vi "SciScan GALVO.vi"(11 "System type (Default - Standalone)":T1(ring)) -> ()   [LabVIEW 2012]
doc: "SciScan 1.1f2 160418"
uses:
  Custom Controls/Laser power 2 dial.ctl
  Custom Controls/Ch selector.ctl
  Custom Controls/MAIN Image panel tab Control type def.ctl
  Custom Controls/scan mode main settings tab.ctl
  Custom Controls/speed mode type def.ctl
  Custom Controls/pixel resolution enum.ctl
  Custom Controls/advanced settings inner tab CTL.ctl
  Custom Controls/Laser power 1 dial.ctl
  Custom Controls/Histogram tab.ctl
  Custom Controls/file format type def.ctl
  Custom Controls/experiment type.ctl
  Custom Controls/display palette control.ctl
  Custom Controls/PositionSaveMod.ctl
  Custom Controls/trigger enum.ctl
  HFG/Custom Controls and Typedefs/HFG Commands.ctl
  CommonResource VIs/Timing/Timer Commands.ctl
  HFG/SubVIs/Broken Chain FGV Command.ctl
  Plugins/Macro Module/Macro Rule/subVIs/MacroRules_FGV_Commands.ctl
  Plugins/Macro Module/Macro Rule/subVIs/MacroErrorsFGV_Commands.ctl
  <vilib>/event_ctls.llb/lveventtype.ctl
  INI/settingsIO/Settings IO_Commands.ctl
  Plugins/Macro Module/MacroGUI Module/Custom Controls and Typedefs/GFG Variable for IO.ctl
  GFG/GFGnumericGet.vi
  GFG/GFGfpRefGet.vi
  GFG/GFGpathGet.vi
  GFG/GFGstringGet.vi
  GFG/GFG library.lvlib
panel:
  in  "MAIN UI responsive? (F)":bool
  in  "shutterlock":bool caption="LOCK"
  in  "custom step z":bool
  in  "custom step xy":bool
  in  "no of grid lines":dbl(slide) min=0.0 step=1.0 scale=0.0..20.0
  out "grid size":string caption="GRID"
  in  "save prot":bool
  in  "piezo.active":bool
  in  "PositionSaveButton":T2
  in  "reset zoom":bool
  out "Channel 5 large":T3(plugin-control)
  in  "bool.stage.speed":bool=TRUE
  in  "Stage Stop":bool
  in  "step.size.xy":u16(ring)=1 items=["   1"=1, "   2"=2, "   5"=5, "  10"=10, "  20"=20, "  50"=50, "100"=100]
  in  "Y UP":bool
  in  "X LEFT":bool
  in  "Y DOWN":bool
  in  "X RIGHT":bool
  out "String 6":string
  in  "shutter":bool
  in  "x.pixels":i32=256 min=2 max=2048 step=2
  in  "clear prot":bool
  in  "timestamp.prot":bool
  in  "protocol.notes":string caption="notebook"
  in  "Open All\nSettings":bool=TRUE
  in  "step.size.z":u16(ring)=1 items=["    1"=1, "    2"=2, "    5"=5, "  10"=10, "  20"=20, "  50"=50, "100"=100]
  out "frame count":dbl(slide) scale=0.0..30.0
  in  "scan mode main settings":T4
  in  "pixel resolution":T5=enum."512 x 512"
  in  "speed mode":T6=2 items=["extra fast scan", "fast scan", "standard scan", "long exposure"]
  in  "ROTATE":dbl(knob) min=0.0 max=360.0 step=1.0 scale=0.0..360.0 scale format="%#_3g"
  in  "rotate.enable":bool
  in  "ZOOM":dbl(slide)=1.0 min=1.0 max=20.1 step=0.1 scale=1.0..20.0 scale format="%#.1f"
  in  "no. of frames to acquire":i32=10000 min=2 max=2147483646 step=2
  out "x.fov":dbl caption="Field of view    x" format="%#_3p"
  out "y.fov":dbl caption="y" format="%#_3p"
  out "ms.p.line":dbl caption="ms/line" format="%#.2g"
  out "frames.p.sec":dbl caption="frames/s" format="%#.2g"
  out "pixels per line":i32=10000 min=2 max=2147483646 step=2
  out "lines per second":i32=10000 min=2 max=2147483646 step=2
  in  "linescan.y.pixels":i32=256 caption="Lines to display at once" min=2 max=2048 step=2
  in  "no. of lines to acquire":i32=10000 min=2 max=2147483646 step=2
  in  "experiment type":T7="XYT"
  in  "experiment name":string
  in  "root.path":path=path "d:/"
  in  "Objective":u16(ring) items=["Olympus 10x", "Nikon 20x", "Nikon 16x"]
  in  "file format":T8
  out "stack.duration":i32=10 caption="stack.duration (sec)" min=0 max=2147483646 step=2
  in  "add":bool
  in  "clear all":bool
  in  "clear last":bool
  in  "move to z.stack.\nstart plane":bool
  in  "start z.stack":bool
  in  "frames.per.plane":i32=10000 min=2 step=2
  in  "z.spacing":dbl=1.0 caption="z.spacing (um)" min=0.1 step=0.1
  out "no of planes":i32=10 min=0 max=2147483646 step=2
  in  "no.of.cycles.to.scan":dbl=2.0 caption="no.of.volumes" min=1.0 step=1.0
  out "volume rate (in Hz)":dbl=1.0 min=0.0 max=5.5 step=0.1
  in  "frames.per.z.cycle":dbl=4.0 min=4.0 step=2.0
  in  "piezo.mode":bool
  in  "piezo.offset.compensation.seconds":dbl caption="no.of.volumes"
  in  "Z UP":bool
  in  "Z DOWN":bool
  out "String 7":string
  in  "setY":dbl caption="Z-Stepper" format="%#.1f"
  in  "setX":dbl caption="Z-Stepper" format="%#.1f"
  in  "setZ":dbl caption="set" format="%#.1f"
  out "String 4":string
  out "posZ":dbl caption="actual" format="%#.1f"
  out "posX":dbl caption="Z-Stepper" format="%#.1f"
  out "posY":dbl caption="Z-Stepper" format="%#.1f"
  out "String 3":string
  in  "XYZ stage settings slider tab":enum32{" "}(tab)
  in  "LP enable":bool
  out "String 20":string
  in  "set stage speed":bool
  in  "enable virtual XYZ":bool
  out "String 16":string
  in  "set Y to zero":bool
  in  "set X to zero":bool
  in  "set all to zero":bool
  in  "set Z to zero":bool
  out "String 9":string
  in  "reverse x":bool
  in  "reverse y":bool
  in  "reverse z":bool
  out "String 8":string
  in  "PIN Button XYZ stage settings slider tab":bool=TRUE
  in  "QUIT":bool
  in  "Record":bool
  in  "FOCUS":bool
  in  "MAIN Image panels":T9
  out "Channel 1 large":T3(plugin-control)
  out "Channel 2 large":T3(plugin-control)
  out "Channel 3 large":T3(plugin-control)
  out "Channel 4 large":T3(plugin-control)
  out "Channel 1 small":T3(plugin-control)
  out "Channel 2 small":T3(plugin-control)
  out "Channel 4 small":T3(plugin-control)
  out "Channel 3 small":T3(plugin-control)
  in  "Blue Channel (Overlay)":T10 caption="B"
  in  "Green Channel (Overlay)":T10=enum."Ch 1" caption="G"
  in  "Red Channel (Overlay)":T10=enum."Ch 2" caption="R"
  out "RGB overlay":T3(plugin-control)
  in  "ROI channel":T10=enum."Ch 1" caption="Channel"
  out "ROI chart":sgl[][](graph)=[[54.570076, 54.556858]]
  out "ROI Image display":T3(plugin-control)
  in  "zoom to ROI":bool
  in  "move.to.point.ROI":bool
  in  "load coordinates":bool
  in  "confirm line":bool
  in  "channel arb line scan":T10 caption="Channel"
  out "arb line scan display":T3(plugin-control)
  in  "Cancel":bool
  in  "hist/ref slider tab":enum32{" "}(tab)
  in  "PIN Button hist/ref slider tab":bool=TRUE
  in  "Histograms tab":T11
  in  "auto scale\n      CH 1":bool=TRUE caption="auto scale 2"
  in  "Min Max Channel 1":cluster{dbl, dbl}(slide)={0.0, 2047.0} scale=0.0..2047.0 scale format="%#_4g"
  out "Histogram 1":T12(graph)={"Starting Value"=-2007.0, "Incremental Value"=15.7109375, "Histogram"=[]}
  out "String 12":string
  in  "auto scale\n      CH 4":bool=TRUE caption="auto scale 2"
  in  "Min Max Channel 4":cluster{dbl, dbl}(slide)={0.0, 2047.0} scale=0.0..2047.0 scale format="%#_4g"
  out "Histogram 4":T12(graph)
  out "String 15":string
  in  "auto scale\n      CH 3":bool=TRUE caption="auto scale 2"
  in  "Min Max Channel 3":cluster{dbl, dbl}(slide)={0.0, 2047.0} scale=0.0..2047.0 scale format="%#_4g"
  out "Histogram 3":T12(graph)
  out "String 14":string
  in  "auto scale\n      CH 2":bool=TRUE caption="auto scale 2"
  in  "Min Max Channel 2":cluster{dbl, dbl}(slide)={0.0, 2047.0} scale=0.0..2047.0 scale format="%#_4g"
  out "Histogram 2":T12(graph)
  out "String 13":string
  in  "avg type":u16(ring) items=["none", "group avg", "moving avg"]
  in  "avg of":i8=10 min=2 step=1
  in  "display palette":T13
  in  "large histogram":bool caption="Pop-Out"
  in  "laser power slider tab":enum32{"1", " 2"}(tab)
  in  "enable set power max":bool
  in  "set power max":bool
  in  "Laser Power":T14 min=0.0 max=100.0 step=0.5 scale=0.0..100.0 scale format="%3d"
  in  "PIN Button laser power slider tab":bool=TRUE
  in  "enable set power max 2":bool
  in  "set power max 2":bool
  in  "Laser Power 2":T15 caption="Laser Power" min=0.0 max=100.0 step=0.5 scale=0.0..100.0 scale format="%3d"
  in  "PMT slider tab":enum32{""}(tab)
  in  "PMT 2":u16(slide) max=1000 scale=0.0..1000.0
  in  "PMT 1":u16(slide) max=1250 scale=0.0..1000.0
  out "String 5":string
  in  "PMT 4":u16(slide) max=1000 scale=0.0..1000.0
  in  "PMT 3":u16(slide) max=1250 scale=0.0..1000.0
  out "String 18":string
  in  "PIN Button PMT slider tab":bool=TRUE
  in  "advanced settings slider tab":enum32{""}(tab)
  in  "advanced settings inner tab":T16
  in  "pixel.dwell.time.in.sec":dbl=1e-05 min=4e-07 max=1e-05 step=2e-07 format="%#.6p"
  in  "y.pixel.sz":dbl=1e-05 min=1e-09 max=1e-05 step=1e-07 format="%#_3p"
  in  "x.pixel.sz":dbl=1e-05 min=1e-09 max=1e-05 step=1e-07 format="%#_3p"
  in  "y.pixels":i32=512 caption="Y Resolution" min=2 max=2048 step=2
  in  "fill fraction":dbl=60.0 caption="%" min=60.0 max=100.0 step=0.5 format="%_3g"
  in  "nomin.x.pixels":i32=512 caption="X resolution" min=2 max=2048 step=2
  in  "y bidirectional":bool
  in  "x bidirectional":bool=TRUE
  in  "x.voltage":dbl=0.9999999999999999 min=0.0 max=5.5 step=0.1
  in  "y.voltage":dbl=1.0 min=0.0 max=5.5 step=0.1
  in  "y.volt.offset":dbl=-0.2 step=0.1
  in  "x.volt.offset":dbl=-0.2 step=0.1
  in  "voltage.for\nmax.field.of.view":dbl=5.0 min=0.0 max=5.0
  in  "max.field.of.view":dbl=300.0 format="%#_6p"
  in  "x.invert.image":bool
  in  "y.invert.image":bool
  in  "autocorrect.startdelay":bool
  out "pixel.dwell.time.in.ticks":u16=20 min=2 step=1
  out "sample.clock":dbl=5000000.0
  out "ADsamples.per.frame":i32
  in  "Start.Delay":dbl(slide)=1.0 min=1.0 max=10000000.0 step=1.0 scale=1.0..1000.0
  in  "invert.ch.3":bool
  in  "invert.ch.2":bool
  in  "invert.ch.1":bool
  in  "invert.ch.0":bool caption="invert"
  in  "ai.active3":bool
  in  "ai.active2":bool
  in  "ai.active1":bool
  in  "ai.active0":bool caption="active"
  in  "ai.range2":dbl=10.0 min=0.1 max=10.0 step=0.1
  in  "ai.range1":dbl=10.0 min=0.1 max=10.0 step=0.1
  out "ai.string3":string
  out "ai.string2":string
  out "ai.string1":string
  out "ai.string0":string caption="Analog Input"
  in  "ai.range0":dbl=10.0 caption="input range\n      (+/-)" min=0.1 max=10.0 step=0.1
  in  "ai.range3":dbl=10.0 min=0.1 max=10.0 step=0.1
  in  "Pulse\nevery n frames":i32=2 min=1 max=10000 step=1
  in  "Initial delay\n[frames]":dbl=2.0 min=0.1 step=1.0
  in  "pulse.Boolean":bool
  in  "external.start.trigger.enable":bool=TRUE caption="WAIT FOR TRIGGER from external device"
  in  "trigger.enum":T17=enum."trigger off" caption="SEND TRIGGER to external device"
  in  "Initial delay\n[ms]":dbl=2.0 min=0.1 max=170000.0 step=1.0
  in  "Pulse\nduration [ms]":dbl=2.0 min=0.1 step=1.0
  in  "Pulse\nfrequency [Hz]":dbl=2.0 min=0.01 max=10000.0 step=1.0
  in  "abs/rel z pos":enum32{"abs", "rel"}(tab)
  in  "pos  pockels cell PMT Data":dbl[][](array[numeric]) caption="Data" format="%0.1f"
  in  "RELATIVE pos  pockels cell PMT Data":dbl[][](array[numeric]) caption="Data" format="%0.1f"
  in  "PIN Button advanced settings slider tab":bool=TRUE
  in  "SCIENTIFICA Button":bool
  # "to zoom out press and hold Shift"
  # "OFF"
  # "2x2"
  # "4x4"
  # "6x6"
  # "8x8"
  # "10x10"
  # "12x12"
  # "14x14"
  # "16x16"
  # "18x18"
  # "20x20"
  # "abs  pos."
  # "x"
  # "y"
  # "z"
  # "rel pos."
  # "x"
  # "y"
  # "z"
  # "Z Stack parameters"
  # "Z Stack plane management"
  # "zig-zag (leaf scan)"
  # "sawtooth"
  # "Typically, the response lag of piezo positioning is in the millisecond range. Use negative values to compensate for this lag.  Example: -0.015 seconds"
  # "reverse \ndirection"
  # "Zero\nrel. pos."
  # "z"
  # "x"
  # "y"
  # "LP enable"
  # "virtual XYZ"
  # "Press and hold Ctrl to add multiple ROIs"
  # "Average frames (display only)"
  # "frames"
  # "ms \nHz"
  # "X"
  # "Y"
  # "Z"
  # "LASER1"
  # "LASER2"
  # "X"
  # "Y"
  # "Z"
  # "LASER1"
  # "LASER2"
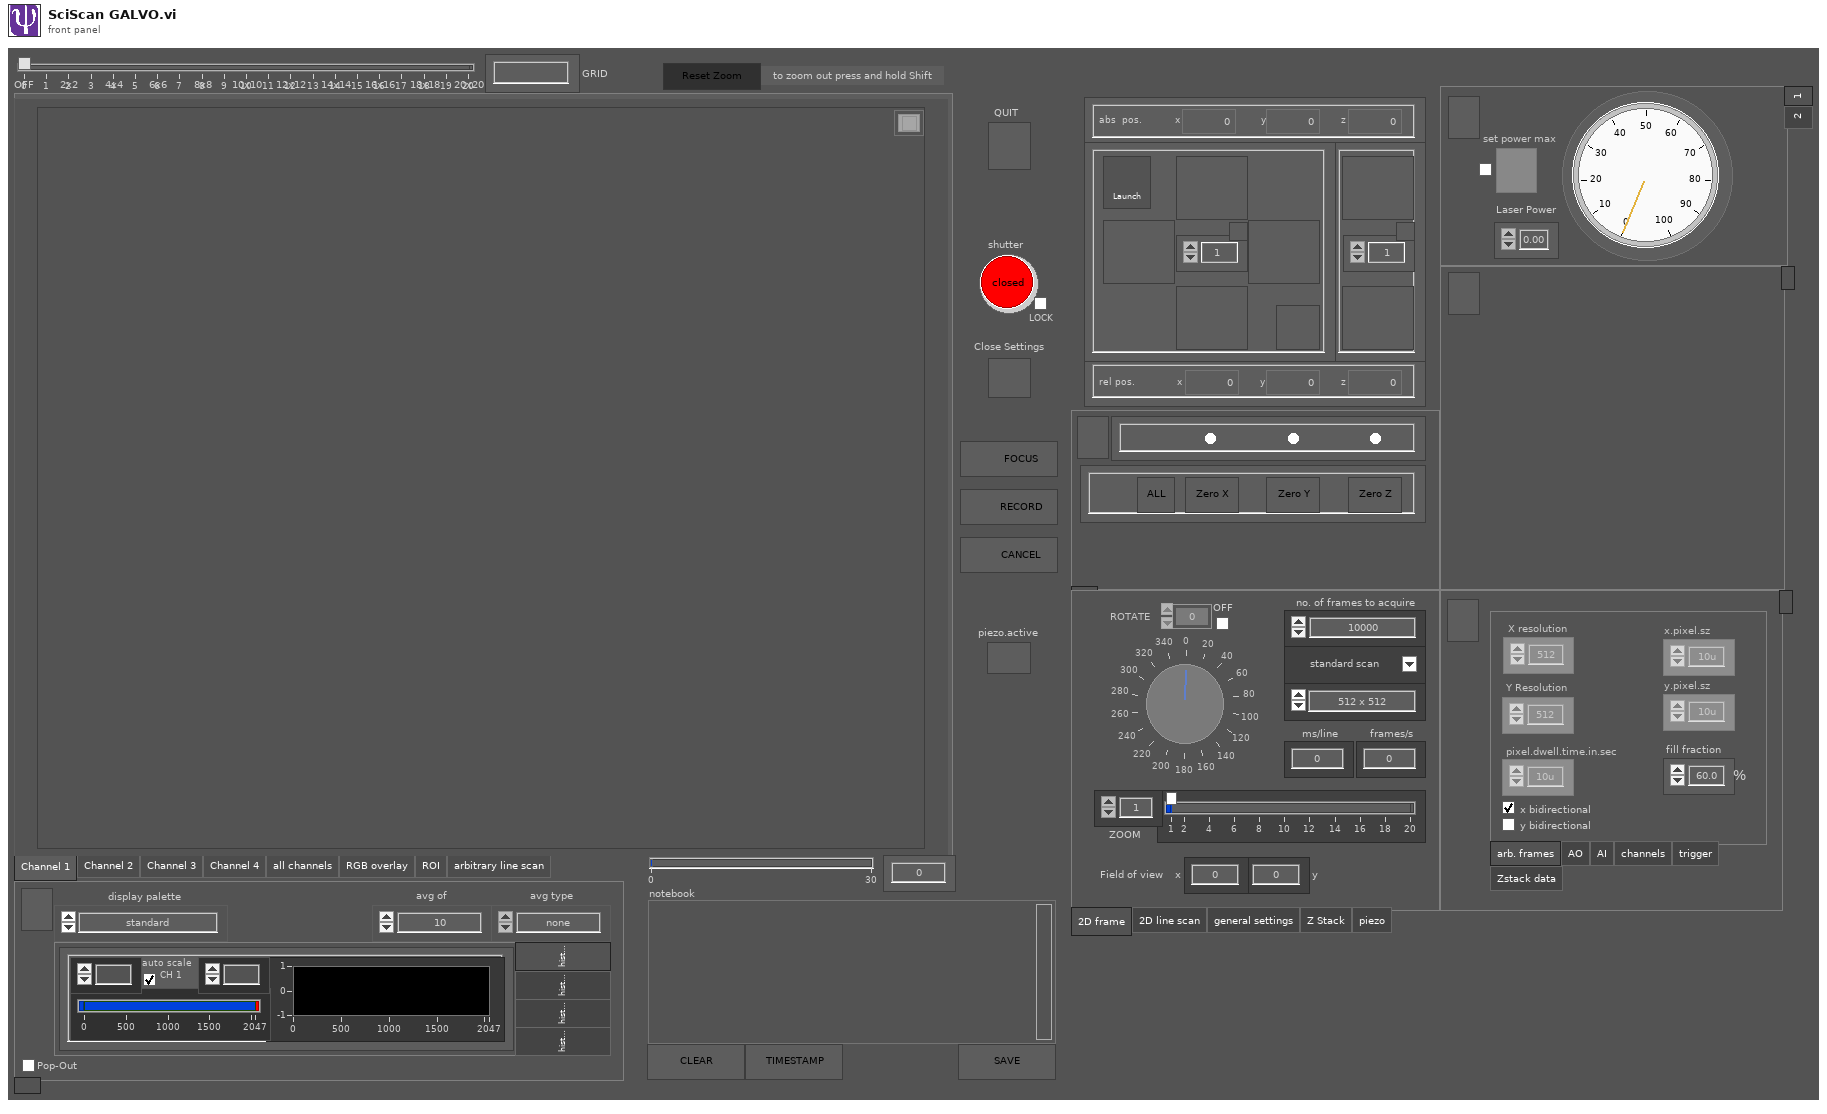
[diagram p1: front panel]
types:
  T1 = enum16{"Standalone Galvo", "Imaging Galvo", "Photostimulation Galvo"}
  T2 = typedef "PositionSaveMod.ctl" = bool
  T3 = typedef "IMAQ Image.ctl" = refnum<image>
  T4 = typedef "scan mode main settings tab.ctl" = enum32{"2D frame", "2D line scan", "general settings", "Z Stack", "piezo"}
  T5 = typedef "pixel resolution enum.ctl" = enum16{"128 x 128", "256 x 128", "256 x 256", "512 x  64", "512 x 128", "512 x 256", "512 x 512", "1024 x 512", "1024 x 1024", "arbitrary"}
  T6 = typedef "speed mode type def.ctl" = u16
  T7 = typedef "experiment type.ctl" = string
  T8 = typedef "file format type def.ctl" = enum16{"16bit raw", "32bit raw", "16bit multi-tiff (interleave)", "16bit multi-tiff (separate)", "16bit multi-tiff (stacked)", "32bit multi-tiff (interleave)", "32bit multi-tiff (separate)", "32bit multi-tiff (stacked)", "16bit tiff series (interleave)", "16bit tiff series (separate)", "16bit tiff series (stacked)", "32bit tiff series (interleave)", "32bit tiff series (separate)", "32bit tiff series (stacked)"}
  T9 = typedef "MAIN Image panel tab Control type def.ctl" = enum32{"Channel 1", "Channel 2", "Channel 3", "Channel 4", "all channels", "RGB overlay", "ROI", "arbitrary line scan"}
  T10 = typedef "Ch selector.ctl" = enum16{"none", "Ch 1", "Ch 2", "Ch 3", "Ch 4"}
  T11 = typedef "Histogram tab.ctl" = enum32{"hist Ch 1", "hist Ch 4", "hist Ch 3", "hist Ch 2"}
  T12 = cluster{"Starting Value":sgl, "Incremental Value":sgl, "Histogram":u32[]}
  T13 = typedef "display palette control.ctl" = enum16{"standard", "high clipping red", "low clipping blue", "high and low clipping", "high / low (full range)"}
  T14 = typedef "Laser power 1 dial.ctl" = dbl
  T15 = typedef "Laser power 2 dial.ctl" = dbl
  T16 = typedef "advanced settings inner tab CTL.ctl" = enum32{"arb. frames", "AO", "AI", "channels", "trigger", "Zstack data"}
  T17 = typedef "trigger enum.ctl" = enum16{"legacy frame pulser PFI4", "continuous pulses", "single pulse", "trigger off"}
  T18 = enum16{"Get Settings Table ", "Read Settings File", "Get Specified Settings"}
  T19 = typedef "MacroErrorsFGV_Commands.ctl" = enum16{"Initialize", "Get Error Array", "Set Error Array"}
  T20 = typedef "MacroRules_FGV_Commands.ctl" = enum16{"Read File", "Get All", "Get Param and Flags"}
  T21 = typedef "Broken Chain FGV Command.ctl" = enum16{"Initialize", "Update VI status", "Get All VI status"}
  T22 = typedef "Timer Commands.ctl" = enum16{"Clear All", "Start", "Pause", "Check Time"}
  T23 = typedef "HFG Commands.ctl" = enum16{"Set", "Get", "Initialize"}
  T24 = enum8{"Enabled", "Disabled", "Disabled and Grayed Out"}
  T25 = typedef "Image Type" = u32
  T26 = cluster{refnum<vi>, refnum<vi>, refnum<vi>, refnum<vi>, refnum<vi>, refnum<vi>, refnum<vi>, refnum<vi>, refnum<vi>, refnum<vi>, refnum<vi>, refnum<vi>}
  T27 = cluster{"New Image":T3, "New Image":T3, "New Image":T3, "New Image":T3, "New Image":T3, "New Image":T3, "New Image":T3, "New Image":T3, "New Image":T3, "New Image":T3, "New Image":T3, "New Image":T3}
  T28 = cluster{"WaveformChartRef":refnum<vi>, "DigitalRef":refnum<vi>, "ArrayRef":refnum<vi>, "TabControlRef":refnum<vi>, "EnumRef":refnum<vi>, "RingRef":refnum<vi>, "BooleanRef":refnum<vi>, "KnobRef":refnum<vi>, "SlideRef":refnum<vi>, "PathRef":refnum<vi>, "StringRef":refnum<vi>, "ComboBox":refnum<vi>, "WaveformGraphRef":refnum<vi>}
  T29 = typedef "lveventtype.ctl" = enum32{"Null", "Timeout", "Annotation Menu Selection", "Annotation Menu Selection?", "App Instance Close", "App Instance Close?", "Autoscale Range Change", "Cell Edit", "Cell Edit?", "Cursor Grab", "Cursor Grab?", "Cursor Menu Selection", "Cursor Menu Selection?", "Cursor Move", "Cursor Release", "Data Change", "Direction Change", "Display State Change", "Drag Ended", "Drag Enter", "Drag Leave", "Drag Over", "Drag Source Update", "Drag Starting", "Drag Starting?", "Drop", "Exec State Change", "Key Down", "Key Down?", "Key Repeat", "Key Repeat?", "Key Up", "Listbox Double Click", "Menu Activation?", "Menu Selection (App)", "Menu Selection? (App)", "Menu Selection (User)", "Mouse Down", "Mouse Down?", "Mouse Enter", "Mouse Leave", "Mouse Move", "Mouse Up", "NI Security User Change (App)", "Pane Size", "Panel Close", "Panel Close?", "Panel Resize", "Plot Attribute Change", "Scale Range Change", "Shortcut Menu Activation?", "Shortcut Menu Selection (App)", "Shortcut Menu Selection? (App)", "Shortcut Menu Selection (User)", "Tree Double Click", "Tree Drag", "Tree Drag?", "Tree Drop", "Tree Drop?", "Tree Item Close", "Tree Item Close?", "Tree Item Open", "Tree Item Open?", "Value Change"}
  T30 = enum32{"Invalid", "Standard", "Closed", "Hidden", "Minimized", "Maximized"}
  T31 = enum32{"Invalid", "Default", "Floating", "Floating/Auto-Hide", "Modal"}
  T32 = typedef "Settings IO_Commands.ctl" = enum16{"Write HW Settings", "Write Config Settings", "Read HW Settings", "Read Config Settings", "Write Line-Scan Settings", "Write Frame-Scan Settings", "Write Z-Stack Settings", "Read Line-Scan Settings", "Read Frame-Scan Settings", "Read Z-Stack Settings", "Read Fast-Z Settings", "Write Fast-Z Settings"}
  T33 = typedef "GFG Variable for IO.ctl" = cluster{"Variable Name":string, "Value (Variant)":variant, "data type":string}
  T34 = enum32{"Page Enabled", "Page Disabled", "Page Disabled & Grayed"}
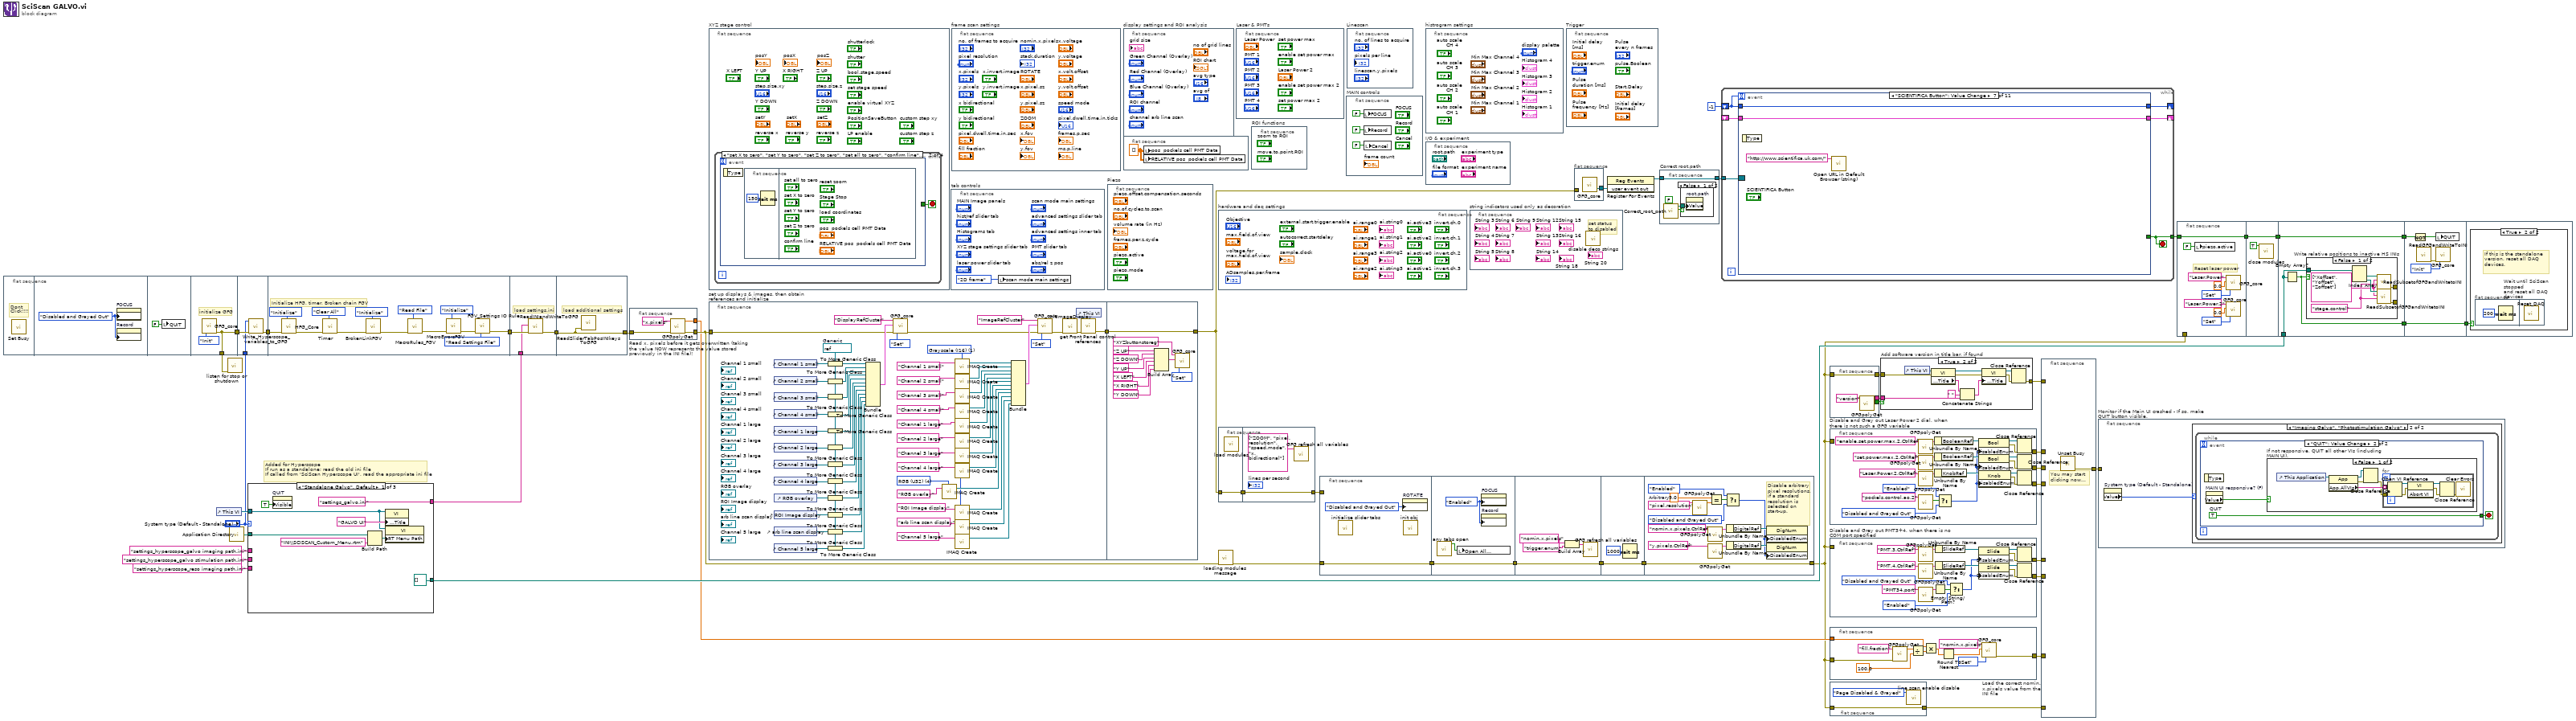
[diagram p0: block diagram]
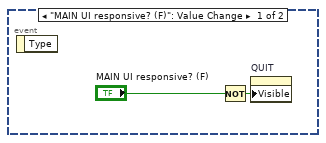
[diagram p3: hidden frame]
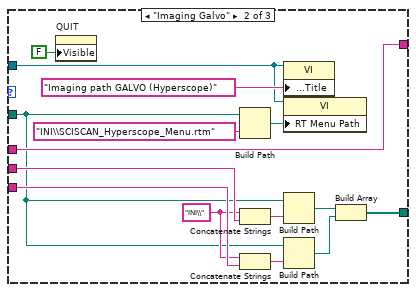
[diagram p6: hidden frame]
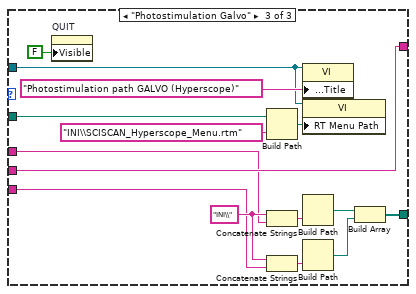
[diagram p7: hidden frame]
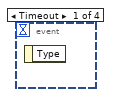
[diagram p9: hidden frame]
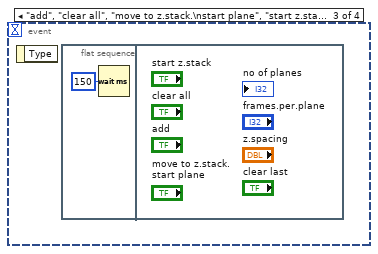
[diagram p10: hidden frame]
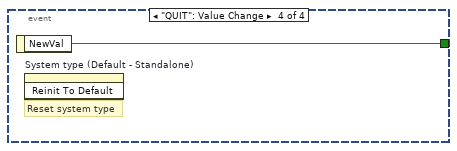
[diagram p11: hidden frame]
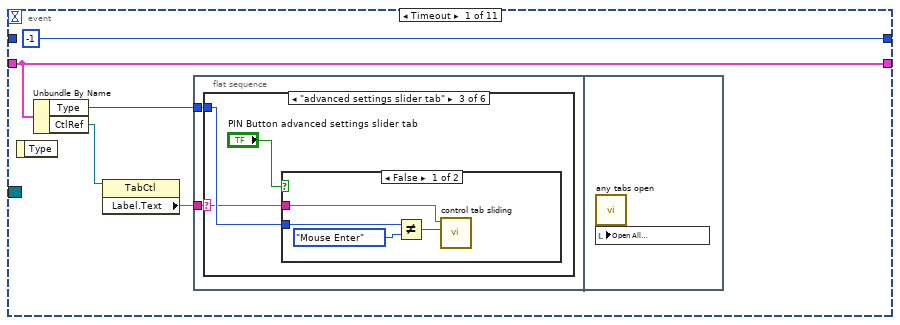
[diagram p14: hidden frame]
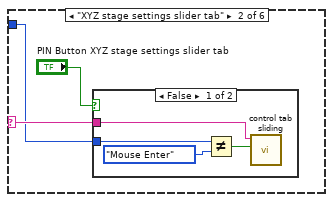
[diagram p16: hidden frame]
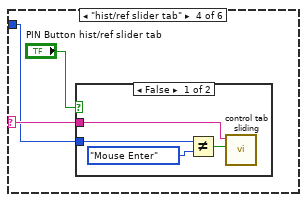
[diagram p19: hidden frame]
diagram:
  # "Added for Hyperscope\nIf run as a standalone; read the old ini file\nIf called from 'SciScan Hyperscope UI', read the appropriate ini file"
  n1 = flat-sequence {
    tunnel: [w51] -> w23
    tunnel: [w51] -> w38
    tunnel: w23 -> [w55]
    tunnel: [w54] -> w22
    tunnel: "System type (Default - Standalone)" -> [w53]
    tunnel: w22 -> [w68]
    tunnel: [w56] -> w48
    tunnel: w48 -> [w71]
    tunnel: [w70] -> w47
    tunnel: w34 -> [w69]
    tunnel: [w72] -> w14
    tunnel: w47 -> [w72]
    frame #0 {
      # "Dont\nClick!!!!"
      n2 = call <vilib>:"Set Busy.vi"() -> ()  [unwired: 10 in, 2 out]
    }
    frame #1 {
      w49 = T24."Disabled and Grayed Out" ("Disabled")
      n3 = property on="FOCUS" class="Bool (strict)"("DisabledEnum"=w49) -> ()  [unwired: 2 in, 2 out]
      n4 = property on="Record" class="Bool (strict)"("DisabledEnum"=w49) -> ()  [unwired: 2 in, 2 out]
    }
    frame #2 {
      n5 = local write "QUIT"(FALSE ("QUIT")) -> ()
    }
    frame #3 {
      # "initialize GFG"
      n6 = call "GFG_core.vi"("Action"=enum16{"Init", "Set", "Get"}."Init") -> ("error out"=w51:errorcluster)  [unwired: 12 in, 6 out]
    }
    frame #4 {
      n7 = call "Write_Hyperscope_variables_to_GFG.vi"("error in (no error)"=w55, "System type (Default - Standalone)"=w53) -> ("error out"=w54:errorcluster)  [unwired: 9 in]
    }
    frame #5 {
      # "Initialize HFG, timer, Broken chain FGV"
      n8 = call "HFG_Core.vi"("HFG Commands"=HFG_Commands."Initialize", "Error In"=w68) -> ("Error Out"=w65:errorcluster)  [unwired: 6 in, 3 out]
      n9 = call "Timer.vi"("Timer Command"=Timer_Commands."Clear All", "Error In"=w65) -> ("Error Out"=w63:errorcluster)  [unwired: 4 in, 5 out]
      n10 = call "BrokenLinkFGV.vi"("Broken Chain FGV Action"=Broken_Chain_FGV_Command."Initialize", "Error In"=w63) -> ("Error Out"=w61:errorcluster)  [unwired: 7 in, 2 out]
      n11 = call "MacroRules_FGV.vi"("MacroRules_FGV_Commands"=MacroRules_FGV_Commands."Read File", "Error In"=w61) -> ("Error Out"=w60:errorcluster)  [unwired: 5 in, 4 out]
      n12 = call "MacroErrorsFGV.vi"("MacroErrorsFGV_Commands"=MacroErrorsFGV_Commands."Initialize", "Error In"=w60) -> ("Error Out"=w58:errorcluster)  [unwired: 8 in, 1 out]
      n13 = call "FGV_Settings IO Rule.vi"("Command_Settings IO Rule"=T18."Read Settings File", "Error In"=w58) -> ("Error Out"=w56:errorcluster)  [unwired: 7 in, 2 out]
    }
    frame #6 {
      # "load settings.ini"
      n14 = call "ReadINIandWriteToGFG.vi"("error in (no error)"=w71, "name or relative path"=w69) -> ("error out"=w70:errorcluster)  [unwired: 9 in]
    }
    frame #7 {
      # "load additional settings"
      n15 = call "ReadSliderTabPosINIkeysToGFG.vi"("error in (no error)"=w72) -> ()  [unwired: 11 in]
    }
  }
  n16 = control-ref of="This VI"() -> (w33:refnum<vi>)
  n17 = call "listen for stop or shutdown.vi"("error in (no error)"=w38) -> ()  [unwired: 9 in, 2 out]
  n18 = call <vilib>:"Application Directory.vi"() -> ("Application Directory"=w32:path)
  n19 = case shown="\"Standalone Galvo\", Default" "System type (Default - Standalone)" {
    tunnel: ["settings_galvo.ini" ("name or relative path") w90 w104] -> w34
    tunnel: w33 -> [w75 w91 w106]
    tunnel: w32 -> [w76 w82 w105]
    tunnel: "settings_hyperscope_galvo imaging path.ini" ("name or relative path") -> [_ w90 w97]
    tunnel: "settings_hyperscope_galvo stimulation path.ini" ("name or relative path") -> [_ w89 w104]
    tunnel: "settings_hyperscope_reso imaging path.ini" -> [_ w84 w98]
    tunnel: [path[] [] w87 w96] -> w17
    frame "Standalone Galvo", Default {
      n20 = property on="QUIT" class="Bool (strict)"("Visible"=TRUE) -> ()  [unwired: 2 in, 2 out]
      n21 = Build Path(base path=w76, name or relative path="INI\\SCISCAN_Custom_Menu.rtm") -> (appended path=w77:path)
      n22 = property class="VI"(reference=w75, "Front Panel.Title"="GALVO UI" ("Front Panel Window:Title")) -> ()  [unwired: 1 in, 2 out]
      n23 = property class="VI"(reference=w75, "RT Menu Path"=w77) -> ()  [unwired: 1 in, 2 out]
    }
    frame "Imaging Galvo" {
      w83 = "INI\\" ("name or relative path")
      n24 = property on="QUIT" class="Bool (strict)"("Visible"=FALSE) -> ()  [unwired: 2 in, 2 out]
      n25 = Build Path(base path=w82, name or relative path="INI\\SCISCAN_Hyperscope_Menu.rtm") -> (appended path=w93:path)
      n26 = Concatenate Strings(w83, w89) -> (w88:string)
      n27 = Concatenate Strings(w83, w84) -> (w86:string)
      n28 = property class="VI"(reference=w91, "Front Panel.Title"="Imaging path GALVO (Hyperscope)" ("Front Panel Window:Title")) -> ()  [unwired: 1 in, 2 out]
      n29 = property class="VI"(reference=w91, "RT Menu Path"=w93) -> ()  [unwired: 1 in, 2 out]
      n30 = Build Path(base path=w82, name or relative path=w88) -> (appended path=w85:path)
      n31 = Build Path(base path=w82, name or relative path=w86) -> (appended path=w81:path)
      n32 = Build Array(w85, w81) -> (w87:path[])
    }
    frame "Photostimulation Galvo" {
      w100 = "INI\\" ("name or relative path")
      n33 = property on="QUIT" class="Bool (strict)"("Visible"=FALSE) -> ()  [unwired: 2 in, 2 out]
      n34 = Build Path(base path=w105, name or relative path="INI\\SCISCAN_Hyperscope_Menu.rtm") -> (appended path=w107:path)
      n35 = Concatenate Strings(w100, w97) -> (w103:string)
      n36 = Concatenate Strings(w100, w98) -> (w102:string)
      n37 = property class="VI"(reference=w106, "Front Panel.Title"="Photostimulation path GALVO (Hyperscope)" ("Front Panel Window:Title")) -> ()  [unwired: 1 in, 2 out]
      n38 = property class="VI"(reference=w106, "RT Menu Path"=w107) -> ()  [unwired: 1 in, 2 out]
      n39 = Build Path(name or relative path=w103) -> (appended path=w101:path)  [unwired: 1 in]
      n40 = Build Path(name or relative path=w102) -> (appended path=w99:path)  [unwired: 1 in]
      n41 = Build Array(w101, w99) -> (w96:path[])
    }
  }
  n42 = flat-sequence "Read x. pixels before it gets overwritten (taking the value NOW represents the value stored previously in the INI file)!" {
    tunnel: w14 -> [w113]
    tunnel: [w112] -> w12
    tunnel: [w111] -> w13
    frame #0 {
      n43 = call-poly "GFGpolyGet.vi"("error in (no error)"=w113, "Variable Name in"="x.pixels") -> ("error out"=w111:errorcluster, "Numeric"=w112:dbl)  [unwired: 7 in, 1 out]
    }
  }
  n44 = flat-sequence "XYZ stage control" {
    frame #0 {
      n45 = while {
        stop <- w115 stop-if-true
        n46 = event shown="[1] \"set X to zero\", \"set Y to zero\", \"set Z to zero\", \"set all to zero\", \"confirm line\", \"Stage Stop\", \"reset zoom\": Value Change" {
          selector: _ -> [_ _ _ _]
          dyn-events: _ -> [_ _ _ _]
          timeout: _ -> [_ _ _ _]
          tunnel: [_ _ _ w118] -> w115
          event Timeout {
            n47 = event-data() -> ()  [unwired: 1 in, 1 out]
          }
          event "set X to zero", "set Y to zero", "set Z to zero", "set all to zero", "confirm line", "Stage Stop", "reset zoom": Value Change {
            n48 = event-data() -> ()  [unwired: 1 in, 1 out]
            n49 = flat-sequence {
              frame #0 {
                n50 = Wait (ms)(milliseconds to wait=u32 150) -> ()  [unwired: 1 out]
              }
              frame #1 {
              }
            }
          }
          event "add", "clear all", "move to z.stack.\nstart plane", "start z.stack", "clear last", "z.spacing", "frames.per.plane", "no of planes": Value Change {
            n51 = event-data() -> ()  [unwired: 1 in, 1 out]
            n52 = flat-sequence {
              frame #0 {
                n53 = Wait (ms)(milliseconds to wait=u32 150) -> ()  [unwired: 1 out]
              }
              frame #1 {
              }
            }
          }
          event "QUIT": Value Change {
            # "Reset system type"
            n54 = event-data() -> ("NewVal"=w118:bool)  [unwired: 1 in]
            n55 = invoke on="System type (Default - Standalone)" class="Enum (strict)" method="Reinit To Default"() -> ()  [unwired: 3 in, 3 out]
          }
        }
      }
    }
  }
  n56 = flat-sequence "set up displays & images, then obtain references and initialize" {
    tunnel: w13 -> [w138]
    tunnel: [w119] -> w46
    tunnel: [w191] -> w19
    tunnel: w46 -> [w191]
    frame #0 {
      w126 = T25 4 items=["Grayscale (U8)", "Grayscale (I16)", "Grayscale (SGL)", "Complex (CSG)", "RGB (U32)", "HSL (U32)", "RGB (U64)", "Grayscale (U16)"] ("Image Type")
      w121 = T25 1 items=["Grayscale (U8)", "Grayscale (I16)", "Grayscale (SGL)", "Complex (CSG)", "RGB (U32)", "HSL (U32)", "RGB (U64)", "Grayscale (U16)"] ("Image Type")
      w123 = refnum<vi> refnum  # Generic
      n57 = control-ref of="Channel 1 small"() -> (w137:refnum<vi>)
      n58 = control-ref of="Channel 2 small"() -> (w136:refnum<vi>)
      n59 = control-ref of="Channel 3 small"() -> (w135:refnum<vi>)
      n60 = control-ref of="Channel 4 small"() -> (w134:refnum<vi>)
      n61 = control-ref of="Channel 1 large"() -> (w133:refnum<vi>)
      n62 = control-ref of="Channel 2 large"() -> (w132:refnum<vi>)
      n63 = control-ref of="Channel 3 large"() -> (w131:refnum<vi>)
      n64 = control-ref of="Channel 4 large"() -> (w130:refnum<vi>)
      n65 = control-ref of="RGB overlay"() -> (w129:refnum<vi>)
      n66 = control-ref of="ROI Image display"() -> (w128:refnum<vi>)
      n67 = control-ref of="arb line scan display"() -> (w127:refnum<vi>)
      n68 = control-ref of="Channel 5 large"() -> (w125:refnum<vi>)
      n69 = To More Generic Class(target class=w123, reference=w137) -> (generic class reference=w178:refnum<vi>)
      n70 = To More Generic Class(target class=w123, reference=w136) -> (generic class reference=w171:refnum<vi>)
      n71 = To More Generic Class(target class=w123, reference=w135) -> (generic class reference=w170:refnum<vi>)
      n72 = To More Generic Class(target class=w123, reference=w134) -> (generic class reference=w169:refnum<vi>)
      n73 = To More Generic Class(target class=w123, reference=w133) -> (generic class reference=w168:refnum<vi>)
      n74 = To More Generic Class(target class=w123, reference=w132) -> (generic class reference=w177:refnum<vi>)
      n75 = To More Generic Class(target class=w123, reference=w131) -> (generic class reference=w176:refnum<vi>)
      n76 = To More Generic Class(target class=w123, reference=w130) -> (generic class reference=w175:refnum<vi>)
      n77 = To More Generic Class(target class=w123, reference=w129) -> (generic class reference=w174:refnum<vi>)
      n78 = To More Generic Class(target class=w123, reference=w128) -> (generic class reference=w173:refnum<vi>)
      n79 = To More Generic Class(target class=w123, reference=w127) -> (generic class reference=w172:refnum<vi>)
      n80 = To More Generic Class(target class=w123, reference=w125) -> (generic class reference=w122:refnum<vi>)
      n81 = Bundle(w178, w171, w170, w169, w168, w177, w176, w175, w174, w173, w172, w122) -> (w181:T26)  [unwired: 1 in]
      n82 = call "GFG_core.vi"("Variable Name in"="DisplayRefCluster", "Variant in"=w181, "error in (no error)"=w138, "Action"=enum16{"Init", "Set", "Get"}."Set") -> ("error out"=w142:errorcluster)  [unwired: 9 in, 6 out]
      n83 = call "IMAQ Create"("Image Name"="RGB overlay", "Image Type"=w126) -> ("New Image"=w162:T3)  [unwired: 3 in, 1 out]
      n84 = call "IMAQ Create"("Image Name"="Channel 1 small", "Image Type"=w121) -> ("New Image"=w154:T3)  [unwired: 3 in, 1 out]
      n85 = call "IMAQ Create"("Image Name"="Channel 2 small", "Image Type"=w121) -> ("New Image"=w155:T3)  [unwired: 3 in, 1 out]
      n86 = call "IMAQ Create"("Image Name"="Channel 3 small", "Image Type"=w121) -> ("New Image"=w156:T3)  [unwired: 3 in, 1 out]
      n87 = call "IMAQ Create"("Image Name"="Channel 4 small", "Image Type"=w121) -> ("New Image"=w157:T3)  [unwired: 3 in, 1 out]
      n88 = call "IMAQ Create"("Image Name"="Channel 1 large", "Image Type"=w121) -> ("New Image"=w158:T3)  [unwired: 3 in, 1 out]
      n89 = call "IMAQ Create"("Image Name"="Channel 2 large", "Image Type"=w121) -> ("New Image"=w159:T3)  [unwired: 3 in, 1 out]
      n90 = call "IMAQ Create"("Image Name"="Channel 3 large", "Image Type"=w121) -> ("New Image"=w160:T3)  [unwired: 3 in, 1 out]
      n91 = call "IMAQ Create"("Image Name"="Channel 4 large", "Image Type"=w121) -> ("New Image"=w161:T3)  [unwired: 3 in, 1 out]
      n92 = call "IMAQ Create"("Image Name"="ROI Image display", "Image Type"=w121) -> ("New Image"=w163:T3)  [unwired: 3 in, 1 out]
      n93 = call "IMAQ Create"("Image Name"="arb line scan display", "Image Type"=w121) -> ("New Image"=w164:T3)  [unwired: 3 in, 1 out]
      n94 = call "IMAQ Create"("Image Name"="Channel 5 large", "Image Type"=w121) -> ("New Image"=w120:T3)  [unwired: 3 in, 1 out]
      n95 = Bundle("New Image"=w154, "New Image"=w155, "New Image"=w156, "New Image"=w157, "New Image"=w158, "New Image"=w159, "New Image"=w160, "New Image"=w161, "New Image"=w162, "New Image"=w163, "New Image"=w164, "New Image"=w120) -> (w166:T27)  [unwired: 1 in]
      n96 = call "GFG_core.vi"("Variable Name in"="ImageRefCluster", "Variant in"=w166, "error in (no error)"=w142, "Action"=enum16{"Init", "Set", "Get"}."Set") -> ("error out"=w141:errorcluster)  [unwired: 9 in, 6 out]
      n97 = call "InitImageDisplay.vi"("error in (no error)"=w141) -> ("error out"=w140:errorcluster)  [unwired: 10 in]
      n98 = control-ref of="This VI"() -> (w139:refnum<vi>)
      n99 = call "get Front Panel control references.vi"("error in (no error)"=w140, "Main VI"=w139) -> ("error out"=w119:errorcluster)  [unwired: 9 in]
    }
    frame #1 {
      n100 = Build Array("Z UP" ("Variable Name in"), "Z DOWN" ("Variable Name in"), "Y UP" ("Variable Name in"), "X LEFT" ("Variable Name in"), "X RIGHT" ("Variable Name in"), "Y DOWN" ("Variable Name in")) -> (w182:string[])
      n101 = call "GFG_core.vi"("Variable Name in"="XYZbuttonstoreg", "Variant in"=w182, "Action"=enum16{"Init", "Set", "Get"}."Set") -> ()  [unwired: 10 in, 7 out]
    }
  }
  n102 = flat-sequence "tab controls" {
    frame #0 {
      n103 = local write "scan mode main settings"(scan_mode_main_settings_tab."2D frame" ("scan mode main settings")) -> ()
    }
  }
  n104 = flat-sequence "frame scan settings" {
    frame #0 {
    }
  }
  n105 = flat-sequence "Piezo" {
    frame #0 {
    }
  }
  n106 = flat-sequence "display settings and ROI analysis" {
    frame #0 {
    }
  }
  n107 = flat-sequence {
    frame #0 {
      w193 = dbl[][] [] ("pos  pockels cell PMT Data")
      n108 = local write "pos  pockels cell PMT Data"(w193) -> ()
      n109 = local write "RELATIVE pos  pockels cell PMT Data"(w193) -> ()
    }
  }
  n110 = flat-sequence "hardware and daq settings" {
    frame #0 {
    }
  }
  n111 = flat-sequence {
    tunnel: w19 -> [w194]
    tunnel: [w194] -> w45
    tunnel: [w196] -> w42
    tunnel: w45 -> [w196]
    frame #0 {
      n112 = call "load modules.vi"() -> ()  [unwired: 12 in]
    }
    frame #1 {
      n113 = call "GFG refresh all variables.vi"("Variables to refresh"=string[] ["ZOOM", "pixel.resolution", "speed.mode", "x.bidirectional"] ("Variables Names In")) -> ()  [unwired: 11 in]
    }
  }
  n114 = call "loading modules message.vi"("error in"=w13) -> ("error out"=w41:errorcluster)  [unwired: 10 in]
  n115 = flat-sequence "Laser & PMTs" {
    frame #0 {
    }
  }
  n116 = flat-sequence "ROI functions" {
    frame #0 {
    }
  }
  n117 = flat-sequence {
    tunnel: w41 -> [w198]
    tunnel: [w198] -> w40
    tunnel: w42 -> [_]
    tunnel: w40 -> [w200]
    tunnel: [w200] -> w37
    tunnel: w37 -> [w205]
    tunnel: [w205] -> w31
    tunnel: w31 -> [w207]
    tunnel: [w207] -> w30
    tunnel: w30 -> [w221]
    tunnel: [w221] -> w4
    frame #0 {
      n118 = call "initialize slider tabs.vi"() -> ()  [unwired: 12 in]
      n119 = property on="ROTATE" class="Knob (strict)"("DisabledEnum"=T24."Disabled and Grayed Out" ("Disabled")) -> ()  [unwired: 2 in, 2 out]
      n120 = call "init obj.vi"() -> ()  [unwired: 12 in]
    }
    frame #1 {
      w201 = T24."Enabled" ("Disabled")
      n121 = call "any tabs open.vi"() -> ("any tabs open?"=w199:bool)  [unwired: 11 in]
      n122 = local write "Open All\nSettings"(w199) -> ()
      n123 = property on="FOCUS" class="Bool (strict)"("DisabledEnum"=w201) -> ()  [unwired: 2 in, 2 out]
      n124 = property on="Record" class="Bool (strict)"("DisabledEnum"=w201) -> ()  [unwired: 2 in, 2 out]
    }
    frame #2 {
      n125 = Build Array("nomin.x.pixels" ("Variable Name in"), "trigger.enum" ("Variable Name in")) -> (w203:string[])
      n126 = call "GFG refresh all variables.vi"("Variables to refresh"=w203) -> ()  [unwired: 11 in]
    }
    frame #3 {
      n127 = Wait (ms)(milliseconds to wait=u32 1000) -> ()  [unwired: 1 out]
    }
    frame #4 {
      w220 = 9.0  # Arbitrary
      # "Disable arbitrary pixel resolutions, if a standard resolution is selected on start-up."
      n128 = call-poly "GFGpolyGet.vi"("Variable Name in"="pixel.resolution") -> ("Numeric"=w219:dbl)  [unwired: 8 in, 2 out]
      n129 = call-poly "GFGpolyGet.vi"("Variable Name in"="nomin.x.pixels.CtrlRef") -> ("output cluster"=w210:T28)  [unwired: 9 in, 1 out]
      n130 = call-poly "GFGpolyGet.vi"("Variable Name in"="y.pixels.CtrlRef") -> ("output cluster"=w212:T28)  [unwired: 9 in, 1 out]
      n131 = Equal?(x=w220, y=w219) -> (x = y?=w217:bool)
      n132 = Select(t=T24."Enabled" ("Disabled"), s=w217, f=T24."Disabled and Grayed Out" ("Disabled")) -> (s? t:f=w208:T24)
      n133 = Unbundle By Name(w210) -> ("DigitalRef"=w209:refnum<vi>)
      n134 = Unbundle By Name(w212) -> ("DigitalRef"=w213:refnum<vi>)
      n135 = property class="DigNum"(reference=w209, "DisabledEnum"=w208) -> ()  [unwired: 1 in, 2 out]
      n136 = property class="DigNum"(reference=w213, "DisabledEnum"=w208) -> ()  [unwired: 1 in, 2 out]
    }
  }
  n137 = flat-sequence "MAIN controls" {
    frame #0 {
      n138 = local write "FOCUS"(FALSE ("FOCUS")) -> ()
      n139 = local write "Record"(FALSE ("Record")) -> ()
      n140 = local write "Cancel"(FALSE ("Cancel")) -> ()
    }
  }
  n141 = flat-sequence "Linescan" {
    frame #0 {
    }
  }
  n142 = flat-sequence "histrogram settings" {
    frame #0 {
    }
  }
  n143 = flat-sequence "I/O & experiment" {
    frame #0 {
    }
  }
  n144 = flat-sequence "string indicators used only as decoration" {
    frame #0 {
      # "set status\nto disabled"
      n145 = call "disable deco strings.vi"() -> ()  [unwired: 11 in, 1 out]
    }
  }
  n146 = flat-sequence "Trigger" {
    frame #0 {
    }
  }
  n147 = flat-sequence {
    tunnel: [w225] -> w39
    tunnel: w19 -> [_]
    frame #0 {
      n148 = call "GFG_core.vi"() -> ("user event out"=w225:refnum<user-event>)  [unwired: 13 in, 6 out]
    }
  }
  n149 = register-events(w39) -> (reference out=w36:refnum<event-registration>)  [unwired: 2 in, 1 out]
  n150 = flat-sequence "Correct root.path" {
    tunnel: w36 -> [w229]
    tunnel: [w229] -> w35
    frame #0 {
      n151 = call "Correct_root_path.vi"("Display warning? (T)"=FALSE) -> ("Path is correct?"=w227:bool, "Resulting path"=w226:path)  [unwired: 8 in, 1 out]
      n152 = case shown="False" w227 {
        tunnel: w226 -> [w230 _]
        frame False {
          n153 = property on="root.path" class="Path"("Value"=w230) -> ()  [unwired: 2 in, 2 out]
        }
        frame True {
        }
      }
    }
  }
  n154 = while {
    tunnel: [w236] -> w44
    shift-right: [w235] -> _
    shift-left: _ -> [w233]
    shift-right: [w234] -> _
    shift-left: -1 -> [w232]
    tunnel: w35 -> [w231]
    stop <- w236 stop-if-true
    n155 = event shown="[6] \"SCIENTIFICA Button\": Value Change" {
      selector: w231 -> [_ _ _ _ _ _ _ _ _ _ _]
      dyn-events: _ -> [_ _ _ _ _ _ _ _ _ _ _]
      timeout: w232 -> [_ _ _ _ _ _ _ _ _ _ _]
      tunnel: [_ _ "QUIT" w305 _ _ _ _ _ _ _] -> w236
      tunnel: [w237 w280 w289 w304 _ w337 w450 w453 w461 w477 _] -> w235
      tunnel: [-1 w281 w297 -1 _ w338 w451 w454 w464 w478 _] -> w234
      tunnel: w233 -> [w237 w280 w289 w304 _ w337 w450 w453 w460 w477 _]
      tunnel: w232 -> [_ w281 w297 _ _ w338 w451 w454 w463 w478 _]
      event Timeout {
        n156 = event-data() -> ()  [unwired: 1 in, 1 out]
        n157 = Unbundle By Name(w237) -> ("Type"=w239:T29, "CtlRef"=w241:refnum<vi>)
        n158 = property class="TabCtl"(reference=w241) -> ("Label.Text"=w240:string)  [unwired: 1 in, 2 out]
        n159 = flat-sequence {
          tunnel: w240 -> [w243]
          tunnel: w239 -> [w242]
          frame #0 {
            n160 = case shown="\"advanced settings slider tab\"" w243 {
              selector: w243 -> [_ w245 w251 w260 w265 w274]
              tunnel: w242 -> [_ w244 w252 w258 w266 w273]
              frame "False", Default {
              }
              frame "XYZ stage settings slider tab" {
                n161 = case shown="False" "PIN Button XYZ stage settings slider tab" {
                  tunnel: w245 -> [w250 _]
                  tunnel: w244 -> [w249 _]
                  frame False {
                    n162 = Not Equal?(x=w249, y=lveventtype."Mouse Enter" ("Type")) -> (x != y?=w248:bool)
                    n163 = call "control tab sliding.vi"("close(T)/open(F)"=w248, "String"=w250) -> ()  [unwired: 10 in]
                  }
                  frame True {
                  }
                }
              }
              frame "advanced settings slider tab" {
                n164 = case shown="False" "PIN Button advanced settings slider tab" {
                  tunnel: w251 -> [w257 _]
                  tunnel: w252 -> [w256 _]
                  frame False {
                    n165 = Not Equal?(x=w256, y=lveventtype."Mouse Enter" ("Type")) -> (x != y?=w255:bool)
                    n166 = call "control tab sliding.vi"("close(T)/open(F)"=w255, "String"=w257) -> ()  [unwired: 10 in]
                  }
                  frame True {
                  }
                }
              }
              frame "hist/ref slider tab" {
                n167 = case shown="False" "PIN Button hist/ref slider tab" {
                  tunnel: w260 -> [w264 _]
                  tunnel: w258 -> [w263 _]
                  frame False {
                    n168 = Not Equal?(x=w263, y=lveventtype."Mouse Enter" ("Type")) -> (x != y?=w262:bool)
                    n169 = call "control tab sliding.vi"("close(T)/open(F)"=w262, "String"=w264) -> ()  [unwired: 10 in]
                  }
                  frame True {
                  }
                }
              }
              frame "laser power slider tab" {
                n170 = case shown="False" "PIN Button laser power slider tab" {
                  tunnel: w265 -> [w271 _]
                  tunnel: w266 -> [w270 _]
                  frame False {
                    n171 = Not Equal?(x=w270, y=lveventtype."Mouse Enter" ("Type")) -> (x != y?=w269:bool)
                    n172 = call "control tab sliding.vi"("close(T)/open(F)"=w269, "String"=w271) -> ()  [unwired: 10 in]
                  }
                  frame True {
                  }
                }
              }
              frame "PMT slider tab" {
                n173 = case shown="False" "PIN Button PMT slider tab" {
                  tunnel: w274 -> [w278 _]
                  tunnel: w273 -> [w277 _]
                  frame False {
                    n174 = Not Equal?(x=w277, y=lveventtype."Mouse Enter" ("Type")) -> (x != y?=w276:bool)
                    n175 = call "control tab sliding.vi"("close(T)/open(F)"=w276, "String"=w278) -> ()  [unwired: 10 in]
                  }
                  frame True {
                  }
                }
              }
            }
          }
          frame #1 {
            n176 = call "any tabs open.vi"() -> ("any tabs open?"=w279:bool)  [unwired: 11 in]
            n177 = local write "Open All\nSettings"(w279) -> ()
          }
        }
      }
      event "Open All\nSettings": Value Change {
        n178 = event-data() -> ()  [unwired: 1 in, 1 out]
        n179 = case shown="True" "Open All\nSettings" {
          frame False {
            n180 = call "slider tabs open.vi"("close(T)/open(F)"=TRUE) -> ()  [unwired: 11 in]
          }
          frame True {
            n181 = call "slider tabs open.vi"("close(T)/open(F)"=FALSE) -> ()  [unwired: 11 in]
          }
        }
      }
      event "QUIT": Value Change {
        w285 = 0.0
        n182 = event-data() -> ()  [unwired: 1 in, 1 out]
        n183 = call "getVIname.vi"() -> ("VI name"=w296:string)  [unwired: 19 in]
        n184 = call "SendShutdownCommand.vi"("Source VI"=w296) -> ()  [unwired: 11 in]
        n185 = call "GFG_core.vi"("Variable Name in"="shutter", "Variant in"=FALSE ("QUIT"), "Action"=enum16{"Init", "Set", "Get"}."Set") -> ()  [unwired: 10 in, 7 out]
        n186 = call "GFG_core.vi"("Variable Name in"="Cancel", "Variant in"=FALSE ("QUIT"), "Action"=enum16{"Init", "Set", "Get"}."Set") -> ()  [unwired: 10 in, 7 out]
        n187 = local write "Laser Power"(w285) -> ()
        n188 = local write "Laser Power 2"(w285) -> ()
        n189 = Build Array("Laser Power 2" ("Variable Name in"), "Laser Power" ("Variable Name in")) -> (w286:string[])
        n190 = for {
          tunnel: w286 -> [w299] mode=indexing
          n191 = call "GFG_core.vi"("Variable Name in"=w299, "Variant in"=0, "Action"=enum16{"Init", "Set", "Get"}."Set") -> ()  [unwired: 10 in, 7 out]
        }
      }
      event User Event {
        n192 = event-data() -> ("Variable Name"=w302:string, "Variant"=w306:variant)  [unwired: 1 in, 1 out]
        n193 = case shown="\"QUIT\"" w302 {
          tunnel: w306 -> [_ _ w309]
          tunnel: [_ _ w307] -> w305
          frame "False", Default {
          }
          frame "root.path" {
            # "Correct root.path"
            n194 = call "Correct_root_path.vi"() -> ()  [unwired: 9 in, 3 out]
          }
          frame "QUIT" {
            n195 = Variant To Data(type=TRUE ("close FP?"), Variant=w309) -> (data=w307:bool)  [unwired: 1 in, 1 out]
            n196 = property on="QUIT" class="Bool (strict)"("Val(Sgnl)"=w307) -> ()  [unwired: 2 in, 2 out]
          }
        }
      }
      event "large histogram": Value Change {
        n197 = event-data() -> ()  [unwired: 1 in, 1 out]
        n198 = Current VI's Path() -> (path=w311:path)
        n199 = Strip Path(path=w311) -> (stripped path=w316:path)  [unwired: 1 out]
        n200 = Strip Path(path=w316) -> (stripped path=w317:path)  [unwired: 1 out]
        n201 = Build Path(base path=w317, name or relative path="image & display") -> (appended path=w313:path)
        n202 = Build Path(base path=w313, name or relative path="large_histogram.vi" ("Variable Name in")) -> (appended path=w315:path)
        n203 = case shown="True" "large histogram" {
          tunnel: w315 -> [w328 w335]
          frame True {
            n204 = Open VI Reference(vi path=w328) -> (vi reference=w321:refnum<vi>, error out=w320:errorcluster)  [unwired: 5 in]
            n205 = invoke class="VI" method="Run VI"(reference=w321, error in=w320, "Wait until done"=FALSE, "Auto Dispose Ref"=TRUE ("Auto Dispose Reference")) -> (reference out=w326:refnum<vi>, error out=w322:errorcluster)  [unwired: 1 in, 3 out]
            n206 = invoke class="VI" method="FP.Open"(reference=w326, error in=w322, "Activate"=TRUE ("Activate?"), "State"=T30."Standard") -> (reference out=w318:refnum<vi>, error out=w319:errorcluster)  [unwired: 1 in, 3 out]
            n207 = Close Reference(reference=w318, error in (no error)=w319) -> ()  [unwired: 1 out]
          }
          frame False {
            n208 = Open VI Reference(vi path=w335) -> (vi reference=w332:refnum<vi>, error out=w331:errorcluster)  [unwired: 5 in]
            n209 = invoke class="VI" method="FP.Close"(reference=w332, error in=w331) -> (reference out=w329:refnum<vi>, error out=w330:errorcluster)  [unwired: 1 in, 1 out]
            n210 = invoke class="VI" method="Abort VI"(reference=w329, error in=w330) -> (reference out=w334:refnum<vi>, error out=w333:errorcluster)  [unwired: 1 in, 1 out]
            n211 = Close Reference(reference=w334, error in (no error)=w333) -> ()  [unwired: 1 out]
          }
        }
      }
      event Menu Selection (User) {
        n212 = event-data() -> ("ItemTag"=w336:string)  [unwired: 1 in]
        n213 = case shown="\"Uncaging\"" w336 {
          selector: w336 -> [_ _ _ _ _ _ w415 w423 _ _ _]
          frame Default {
          }
          frame "Help" {
            n214 = call <vilib>:"Open URL in Default Browser (string).vi"("URL"="http://sciscan.scientifica.uk.com/") -> ()  [unwired: 5 in, 2 out]
          }
          frame "Macro Module" {
            n215 = call "get all running vis.vi"() -> ("RunningVIRefs"=w343:refnum<vi>[])  [unwired: 11 in]
            n216 = for {
              tunnel: w343 -> [w360] mode=indexing
              tunnel: "MacroGUI_MD.vi" ("ItemTag") -> [w358]
              tunnel: [w357] -> w341
              tunnel: [w356] -> w340
              stop <- w357 stop-if-true
              n217 = property class="VI"(reference=w360) -> (reference out=w356:refnum<vi>, "Name"=w359:string)  [unwired: 1 in, 1 out]
              n218 = Equal?(x=w358, y=w359) -> (x = y?=w357:bool)
            }
            n219 = case shown="True" w341 {
              tunnel: w340 -> [_ w351]
              frame False {
                n220 = One Button Dialog(message="Missing Plugin") -> ()  [unwired: 1 in, 1 out]
              }
              frame True {
                n221 = property class="VI"(reference=w351, "FP.State"=T30."Standard" ("Front Panel Window:State")) -> (reference out=w350:refnum<vi>, error out=w349:errorcluster)  [unwired: 1 in]
                n222 = property class="VI"(reference=w350, error in=w349, "FP.Behavior"=T31."Default" ("Front Panel Window:Behavior")) -> (reference out=w346:refnum<vi>, error out=w347:errorcluster)
                n223 = Close Reference(reference=w346, error in (no error)=w347) -> ()  [unwired: 1 out]
                n224 = First Call?() -> (First Call?: T/F=w345:bool)
                n225 = case shown="True" w345 {
                  frame False {
                  }
                  frame True {
                    n226 = call "GFG_core.vi"("Variable Name in"="SciScript_MD_first_launch", "Variant in"=TRUE, "Action"=enum16{"Init", "Set", "Get"}."Set") -> ()  [unwired: 10 in, 7 out]
                  }
                }
              }
            }
          }
          frame "Position Save Module" {
            n227 = call "get all running vis.vi"() -> ("RunningVIRefs"=w364:refnum<vi>[])  [unwired: 11 in]
            n228 = for {
              tunnel: w364 -> [w377] mode=indexing
              tunnel: "PositionSave_coMD.vi" ("ItemTag") -> [w373]
              tunnel: [w376] -> w362
              tunnel: [w375] -> w361
              stop <- w376 stop-if-true
              n229 = property class="VI"(reference=w377) -> (reference out=w375:refnum<vi>, "Name"=w374:string)  [unwired: 1 in, 1 out]
              n230 = Equal?(x=w374, y=w373) -> (x = y?=w376:bool)
            }
            n231 = case shown="True" w362 {
              tunnel: w361 -> [_ w371]
              frame False {
                n232 = One Button Dialog(message="Missing Plugin") -> ()  [unwired: 1 in, 1 out]
              }
              frame True {
                n233 = call "refresh source enum.vi"() -> ()  [unwired: 12 in]
                n234 = property class="VI"(reference=w371, "FP.State"=T30."Standard" ("Front Panel Window:State")) -> (reference out=w370:refnum<vi>, error out=w369:errorcluster)  [unwired: 1 in]
                n235 = property class="VI"(reference=w370, error in=w369, "FP.Behavior"=T31."Default" ("Front Panel Window:Behavior")) -> (reference out=w366:refnum<vi>, error out=w367:errorcluster)
                n236 = Close Reference(reference=w366, error in (no error)=w367) -> ()  [unwired: 1 out]
              }
            }
          }
          frame "OME Module" {
            n237 = call "get all running vis.vi"() -> ("RunningVIRefs"=w381:refnum<vi>[])  [unwired: 11 in]
            n238 = for {
              tunnel: w381 -> [w399] mode=indexing
              tunnel: "OME_coMD.vi" ("ItemTag") -> [w395]
              tunnel: [w398] -> w379
              tunnel: [w397] -> w378
              stop <- w398 stop-if-true
              n239 = property class="VI"(reference=w399) -> (reference out=w397:refnum<vi>, "Name"=w396:string)  [unwired: 1 in, 1 out]
              n240 = Equal?(x=w396, y=w395) -> (x = y?=w398:bool)
            }
            n241 = case shown="True" w379 {
              tunnel: w378 -> [_ w390]
              frame False {
                n242 = One Button Dialog(message="Missing Plugin") -> ()  [unwired: 1 in, 1 out]
              }
              frame True {
                n243 = property class="VI"(reference=w390, "FP.State"=T30."Standard" ("Front Panel Window:State")) -> (reference out=w389:refnum<vi>, error out=w388:errorcluster)  [unwired: 1 in]
                n244 = property class="VI"(reference=w389, error in=w388, "FP.Behavior"=T31."Default" ("Front Panel Window:Behavior")) -> (reference out=w385:refnum<vi>, error out=w386:errorcluster)
                n245 = Close Reference(reference=w385, error in (no error)=w386) -> (error out=w384:errorcluster)
                n246 = First Call?() -> (First Call?: T/F=w383:bool)
                n247 = case shown="True" w383 {
                  tunnel: w384 -> [_ _]
                  frame False {
                  }
                  frame True {
                    n248 = disable-structure shown="Disabled" {
                      frame Disabled {
                        n249 = call "GFG_core.vi"("Variable Name in"="OME_MD_first_launch", "Variant in"=TRUE, "Action"=enum16{"Init", "Set", "Get"}."Set") -> ()  [unwired: 10 in, 7 out]
                      }
                      frame Enabled {
                      }
                    }
                  }
                }
              }
            }
          }
          frame "Uncaging" {
            n250 = disable-structure shown="Enabled" {
              disable-tunnel: ["Parallel Uncaging Module\\Uncaging UI\\Uncaging Dual.vi" ("name or relative path") "Plugins\\Photostimulation Module_Single Path\\Photostimulation UI.vi" ("name or relative path")] -> w402
              frame Enabled {
              }
              frame Disabled {
                # "Old single path stimulation UI"
              }
            }
            n251 = call <vilib>:"Application Directory.vi"() -> ("Application Directory"=w403:path)
            n252 = Build Path(base path=w403, name or relative path=w402) -> (appended path=w401:path)
            n253 = Open VI Reference(vi path=w401) -> (vi reference=w404:refnum<vi>)  [unwired: 5 in, 1 out]
            n254 = invoke class="VI" method="FP.Open"(reference=w404) -> (reference out=w405:refnum<vi>, error out=w406:errorcluster)  [unwired: 4 in, 3 out]
            n255 = invoke class="VI" method="Run VI"(reference=w405, error in=w406, "Wait until done"=FALSE ("Wait Until Done")) -> (reference out=w407:refnum<vi>, error out=w408:errorcluster)  [unwired: 2 in, 3 out]
            n256 = Close Reference(reference=w407, error in (no error)=w408) -> (error out=w409:errorcluster)
            n257 = call <vilib>:"Clear Errors.vi"("error in (no error)"=w409) -> ()  [unwired: 6 in, 1 out]
          }
          frame "Load HW Settings" {
            n258 = call "Settings IO.vi"("SettingsFileIO_Commands"=Settings_IO_Commands."Read HW Settings") -> ("Error Out"=w414:errorcluster, "Cancelled?"=w413:bool, "Settings Array OUT"=w412:T33[])  [unwired: 8 in]
            n259 = case shown="False" w413 {
              tunnel: w415 -> [w419 _]
              tunnel: w414 -> [w418 _]
              tunnel: w412 -> [w417 _]
              frame False {
                n260 = call "Dialog Load Settings.vi"("Error In"=w418, "Title Bar String"=w419, "Settings IN"=w417) -> ()  [unwired: 7 in, 2 out]
              }
              frame True {
              }
            }
          }
          frame "Load Config. Settings" {
            n261 = call "Settings IO.vi"("SettingsFileIO_Commands"=Settings_IO_Commands."Read Config Settings") -> ("Error Out"=w422:errorcluster, "Cancelled?"=w421:bool, "Settings Array OUT"=w420:T33[])  [unwired: 8 in]
            n262 = case shown="False" w421 {
              tunnel: w423 -> [w427 _]
              tunnel: w422 -> [w426 _]
              tunnel: w420 -> [w425 _]
              frame False {
                n263 = call "Dialog Load Settings.vi"("Error In"=w426, "Title Bar String"=w427, "Settings IN"=w425) -> ()  [unwired: 7 in, 2 out]
              }
              frame True {
              }
            }
          }
          frame "Save HW Settings" {
            n264 = call "FGV_Settings IO Rule.vi"("Command_Settings IO Rule"=T18."Get Specified Settings", "Settings Type IN"="HW Settings") -> ("Specified Settings (OUT)"=w429:string[])  [unwired: 7 in, 2 out]
            n265 = for {
              tunnel: w429 -> [w434] mode=indexing
              tunnel: [w433] -> w428 mode=indexing
              n266 = call "GFG_core.vi"("Variable Name in"=w434) -> ("Variant Out"=w435:variant)  [unwired: 12 in, 6 out]
              n267 = Bundle By Name(cluster=T33 {"Variable Name"="", "Value (Variant)"=variant, "data type"=""}, "Variable Name"=w434, "Value (Variant)"=w435) -> (w433:T33)
            }
            n268 = call "Settings IO.vi"("SettingsFileIO_Commands"=Settings_IO_Commands."Write HW Settings", "Settings Array IN"=w428) -> ()  [unwired: 7 in, 3 out]
          }
          frame "Save Config. Settings" {
            n269 = call "FGV_Settings IO Rule.vi"("Command_Settings IO Rule"=T18."Get Specified Settings", "Settings Type IN"="Configuration Settings") -> ("Specified Settings (OUT)"=w438:string[])  [unwired: 7 in, 2 out]
            n270 = for {
              tunnel: w438 -> [w443] mode=indexing
              tunnel: [w442] -> w437 mode=indexing
              n271 = call "GFG_core.vi"("Variable Name in"=w443) -> ("Variant Out"=w444:variant)  [unwired: 12 in, 6 out]
              n272 = Bundle By Name(cluster=T33 {"Variable Name"="", "Value (Variant)"=variant, "data type"=""}, "Variable Name"=w443, "Value (Variant)"=w444) -> (w442:T33)
            }
            n273 = call "Settings IO.vi"("SettingsFileIO_Commands"=Settings_IO_Commands."Write Config Settings", "Settings Array IN"=w437) -> ()  [unwired: 7 in, 3 out]
          }
          frame "QUIT" {
            n274 = call-poly "GFGpolyGet.vi"("Variable Name in"="QUIT") -> ("output cluster"=w448:T28)  [unwired: 9 in, 1 out]
            n275 = Unbundle By Name(w448) -> ("BooleanRef"=w447:refnum<vi>)
            n276 = property class="Bool"(reference=w447, "Val(Sgnl)"=TRUE) -> ()  [unwired: 1 in, 2 out]
          }
        }
      }
      event "SCIENTIFICA Button": Value Change {
        n277 = event-data() -> ()  [unwired: 1 in, 1 out]
        n278 = call <vilib>:"Open URL in Default Browser (string).vi"("URL"="http://www.scientifica.uk.com/") -> ()  [unwired: 5 in, 2 out]
      }
      event "rotate.enable": Value Change {
        n279 = event-data() -> ()  [unwired: 1 in, 1 out]
        n280 = Select(t=T24."Enabled" ("Disabled"), s="rotate.enable", f=T24."Disabled and Grayed Out" ("Disabled")) -> (s? t:f=w456:T24)
        n281 = property on="ROTATE" class="Knob (strict)"("DisabledEnum"=w456) -> ()  [unwired: 2 in, 2 out]
      }
      event "XYZ stage settings slider tab", "advanced settings slider tab", "hist/ref slider tab", "PMT slider tab", "laser power slider tab": Mouse Enter; "XYZ stage settings slider tab", "advanced settings slider tab", "hist/ref slider tab", "PMT slider tab", "laser power slider tab": Mouse Leave {
        n282 = event-data() -> ("Type"=w462:T29, "CtlRef"=w459:refnum<vi>)  [unwired: 1 in]
        n283 = case shown="1, Default" w463 {
          tunnel: [0 w470] -> w464
          tunnel: w462 -> [_ w467]
          tunnel: w459 -> [_ w469]
          tunnel: [w465 w468] -> w461
          tunnel: w460 -> [w465 _]
          frame 0 {
          }
          frame 1, Default {
            n284 = Bundle("Type"=w467, "CtlRef"=w469) -> (w468:cluster{"Type":T29, "CtlRef":refnum<vi>})  [unwired: 1 in]
            n285 = case shown="\"Mouse Enter\"" w467 {
              tunnel: [0 150] -> w470
              frame "Mouse Leave", Default {
              }
              frame "Mouse Enter" {
              }
            }
          }
        }
      }
      event "clear prot", "timestamp.prot", "protocol.notes": Value Change {
        n286 = event-data() -> ("CtlRef"=w479:refnum<vi>)  [unwired: 1 in]
        n287 = property class="Ctl"(reference=w479) -> ("Label.Text"=w473:string)  [unwired: 1 in, 2 out]
        n288 = case shown="\"timestamp.prot\"" w473 {
          tunnel: "protocol.notes" -> [w487 w488 _]
          tunnel: [w487 w489 ""] -> w476
          frame "Null", Default {
          }
          frame "timestamp.prot" {
            w495 = "frame.count" ("Variable Name in")
            w498 = "\r"
            n289 = Get Date/Time In Seconds() -> (seconds since 1Jan1904=w491:timestamp)
            n290 = call-poly "GFGpolyGet.vi"("Variable Name in"=w495) -> ("Numeric"=w494:dbl)  [unwired: 8 in, 2 out]
            n291 = Format Date/Time String(time format string (%c)="%Y-%m-%d %H:%M:%S%2u", seconds (now)=w491) -> (date/time string=w493:string)  [unwired: 1 in]
            n292 = Number To Decimal String(number=w494) -> (decimal integer string=w496:string)  [unwired: 1 in]
            n293 = Concatenate Strings(w488, "\n##################\n" ("string"), w493, w498, w495, " " ("string"), w496, w498) -> (w489:string)
          }
          frame "clear prot" {
          }
        }
        n294 = flat-sequence {
          tunnel: w476 -> [w484]
          tunnel: [w486] -> w475
          frame #0 {
            n295 = Wait (ms)(milliseconds to wait=u32 40) -> ()  [unwired: 1 out]
            n296 = control-ref of="protocol.notes"() -> (w486:refnum<vi>)
            n297 = call "GFG_core.vi"("Variable Name in"="protocol.notes", "Variant in"=w484, "Action"=enum16{"Init", "Set", "Get", "Clear"}."Set") -> ()  [unwired: 10 in, 7 out]
          }
        }
        n298 = case shown="\"timestamp.prot\"" w473 {
          frame Default {
          }
          frame "timestamp.prot" {
            n299 = flat-sequence {
              frame #0 {
                n300 = Wait (ms)(milliseconds to wait=u32 100) -> ()  [unwired: 1 out]
              }
              frame #1 {
              }
            }
          }
          frame "clear prot" {
            n301 = flat-sequence {
              frame #0 {
                n302 = Wait (ms)(milliseconds to wait=u32 100) -> ()  [unwired: 1 out]
              }
              frame #1 {
              }
            }
          }
        }
        n303 = call "String Ctl Cursor to End.vi"("String Reference in"=w475) -> ()  [unwired: 10 in, 1 out]
      }
      event "save prot": Value Change {
        w512 = "\\" ("string")
        n304 = event-data() -> ()  [unwired: 1 in, 1 out]
        n305 = flat-sequence {
          frame #0 {
            n306 = Wait (ms)(milliseconds to wait=u32 100) -> ()  [unwired: 1 out]
          }
          frame #1 {
          }
        }
        n307 = Get Date/Time In Seconds() -> (seconds since 1Jan1904=w501:timestamp)
        n308 = call-poly "GFGpolyGet.vi"("Variable Name in"="root.path") -> ("Path"=w517:path)  [unwired: 8 in, 2 out]
        n309 = Path To String(path=w517) -> (string=w514:string)
        n310 = Format Date/Time String(time format string (%c)="%Y_%m_%d\\", seconds (now)=w501) -> (date/time string=w513:string)  [unwired: 1 in]
        n311 = Format Date/Time String(time format string (%c)="%Y%m%d_%H_%M_%S", seconds (now)=w501) -> (date/time string=w500:string)  [unwired: 1 in]
        n312 = Concatenate Strings(w514, w512, w513, w512, w500, ".notes.txt" ("string")) -> (w507:string)
        n313 = Search and Replace String(replace all?=TRUE ("replace all? (F)"), input string=w507, search string="[? < > ; ' , * | \" \\t \\r \\n \\s]+", replace string="_" ("replace string (\"\")")) -> (result string=w511:string)  [unwired: 4 in, 3 out]
        n314 = local read "protocol.notes"() -> (w504:string)
        n315 = String To Path(string=w511) -> (path=w506:path)
        n316 = call "checkandcreatefoldersforfullpath.vi"("Path IN"=w506) -> ("Path OUT"=w505:path)  [unwired: 4 in]
        n317 = Write to Text File(file (use dialog)=w505, text=w504) -> ()  [unwired: 2 in, 3 out]
      }
    }
  }
  n318 = flat-sequence {
    tunnel: [w521] -> w21
    tunnel: [w520] -> w20
    tunnel: w4 -> [w519]
    tunnel: [w519] -> w18
    frame #0 {
      n319 = call-poly "GFGpolyGet.vi"("Variable Name in"="version") -> ("Found/Replaced"=w520:bool, "String"=w521:string)  [unwired: 9 in]
    }
  }
  n320 = flat-sequence "Disable and Grey out Laser Power 2 dial, when there is not such a GFG variable" {
    tunnel: w4 -> [_]
    tunnel: [w525] -> w10
    tunnel: [w524] -> w9
    tunnel: [w523] -> w8
    frame #0 {
      n321 = call-poly "GFGpolyGet.vi"("Variable Name in"="enable.set.power.max.2.CtrlRef") -> ("output cluster"=w530:T28)  [unwired: 9 in, 1 out]
      n322 = call-poly "GFGpolyGet.vi"("Variable Name in"="set.power.max.2.CtrlRef") -> ("output cluster"=w533:T28)  [unwired: 9 in, 1 out]
      n323 = call-poly "GFGpolyGet.vi"("Variable Name in"="Laser.Power.2.CtrlRef") -> ("output cluster"=w542:T28)  [unwired: 9 in, 1 out]
      n324 = call-poly "GFGpolyGet.vi"("Variable Name in"="pockels.control.ao.2") -> ("Found/Replaced"=w544:bool)  [unwired: 9 in, 1 out]
      n325 = Unbundle By Name(w530) -> ("BooleanRef"=w529:refnum<vi>)
      n326 = Unbundle By Name(w533) -> ("BooleanRef"=w534:refnum<vi>)
      n327 = Unbundle By Name(w542) -> ("KnobRef"=w541:refnum<vi>)
      n328 = Select(t=T24."Enabled" ("Disabled"), s=w544, f=T24."Disabled and Grayed Out" ("Disabled")) -> (s? t:f=w526:T24)
      n329 = property class="Bool"(reference=w529, "DisabledEnum"=w526) -> (reference out=w528:refnum<vi>, error out=w527:errorcluster)  [unwired: 1 in]
      n330 = property class="Bool"(reference=w534, "DisabledEnum"=w526) -> (reference out=w535:refnum<vi>, error out=w536:errorcluster)  [unwired: 1 in]
      n331 = property class="Knob"(reference=w541, "DisabledEnum"=w526) -> (reference out=w538:refnum<vi>, error out=w537:errorcluster)  [unwired: 1 in]
      n332 = Close Reference(reference=w528, error in (no error)=w527) -> (error out=w525:errorcluster)
      n333 = Close Reference(reference=w535, error in (no error)=w536) -> (error out=w524:errorcluster)
      n334 = Close Reference(reference=w538, error in (no error)=w537) -> (error out=w523:errorcluster)
    }
  }
  n335 = flat-sequence "Disable and Grey out PMT3+4, when there is no COM port specified" {
    tunnel: w4 -> [_]
    tunnel: [w547] -> w7
    tunnel: [w546] -> w6
    frame #0 {
      n336 = call-poly "GFGpolyGet.vi"("Variable Name in"="PMT.3.CtrlRef") -> ("output cluster"=w552:T28)  [unwired: 9 in, 1 out]
      n337 = call-poly "GFGpolyGet.vi"("Variable Name in"="PMT.4.CtrlRef") -> ("output cluster"=w561:T28)  [unwired: 9 in, 1 out]
      n338 = call-poly "GFGpolyGet.vi"("Variable Name in"="PMT34.port") -> ("String"=w549:string)  [unwired: 9 in, 1 out]
      n339 = Empty String/Path?(string/path=w549) -> (empty?=w548:bool)
      n340 = Unbundle By Name(w552) -> ("SlideRef"=w553:refnum<vi>)
      n341 = Unbundle By Name(w561) -> ("SlideRef"=w560:refnum<vi>)
      n342 = Select(t=T24."Disabled and Grayed Out" ("Disabled"), s=w548, f=T24."Enabled" ("Disabled")) -> (s? t:f=w550:T24)
      n343 = property class="Slide"(reference=w553, "DisabledEnum"=w550) -> (reference out=w554:refnum<vi>, error out=w555:errorcluster)  [unwired: 1 in]
      n344 = property class="Slide"(reference=w560, "DisabledEnum"=w550) -> (reference out=w557:refnum<vi>, error out=w556:errorcluster)  [unwired: 1 in]
      n345 = Close Reference(reference=w554, error in (no error)=w555) -> (error out=w547:errorcluster)
      n346 = Close Reference(reference=w557, error in (no error)=w556) -> (error out=w546:errorcluster)
    }
  }
  n347 = flat-sequence "Load the correct nomin.x.pixels value from the INI file" {
    tunnel: w12 -> [w568]
    tunnel: w4 -> [w567]
    tunnel: [w566] -> w5
    frame #0 {
      n348 = call-poly "GFGpolyGet.vi"("error in (no error)"=w567, "Variable Name in"="fill.fraction") -> ("Numeric"=w572:dbl)  [unwired: 7 in, 2 out]
      n349 = Divide(x=w572, y=100.0) -> (x/y=w573:dbl)
      n350 = Multiply(x=w568, y=w573) -> (x*y=w565:dbl)
      n351 = Round To Nearest(number=w565) -> (nearest integer value=w564:dbl)
      n352 = call "GFG_core.vi"("Variable Name in"="nomin.x.pixels", "Variant in"=w564, "Action"=enum16{"Init", "Set", "Get", "Clear"}."Set") -> ("error out"=w566:errorcluster)  [unwired: 10 in, 6 out]
    }
  }
  n353 = flat-sequence {
    tunnel: w4 -> [w575]
    tunnel: [w575] -> w3
    frame #0 {
      n354 = call "line scan enable disable.vi"("Page Enabled State"=T34."Page Disabled & Grayed") -> ()  [unwired: 11 in]
    }
  }
  n355 = case "Add software version in title bar, if found" shown="True" w20 {
    tunnel: w18 -> [w577 w580]
    tunnel: w21 -> [_ w579]
    tunnel: [w577 w578] -> w11
    frame False {
    }
    frame True {
      n356 = control-ref of="This VI"() -> (w588:refnum<vi>)
      n357 = property class="VI"(reference=w588, error in=w580) -> (reference out=w584:refnum<vi>, error out=w583:errorcluster, "Front Panel.Title"=w587:string)
      n358 = Concatenate Strings(w587, " " ("string"), w579) -> (w585:string)
      n359 = property class="VI"(reference=w584, error in=w583, "Front Panel.Title"=w585) -> (reference out=w582:refnum<vi>, error out=w581:errorcluster)
      n360 = Close Reference(reference=w582, error in (no error)=w581) -> (error out=w578:errorcluster)
    }
  }
  n361 = flat-sequence {
    tunnel: w11 -> [_]
    tunnel: w10 -> [_]
    tunnel: w9 -> [_]
    tunnel: w8 -> [_]
    tunnel: w7 -> [_]
    tunnel: w6 -> [_]
    tunnel: w5 -> [_]
    tunnel: w3 -> [_]
    tunnel: [w589] -> w1
    frame #0 {
      # "You may start clicking now..."
      n362 = call <vilib>:"Unset Busy.vi"() -> ("error out"=w589:errorcluster)  [unwired: 11 in]
    }
  }
  n363 = flat-sequence "Monitor if the Main UI crashed - If so, make QUIT button visible." {
    tunnel: w1 -> [_]
    frame #0 {
      n364 = property on="System type (Default - Standalone)" class="Enum (strict)"() -> ("Value"=w590:T1)  [unwired: 2 in, 2 out]
      n365 = case shown="\"Imaging Galvo\", \"Photostimulation Galvo\"" w590 {
        frame "Standalone Galvo", Default {
          # "There is no MAIN UI. Do nothing."
        }
        frame "Imaging Galvo", "Photostimulation Galvo" {
          n366 = while {
            stop <- w591 stop-if-true
            n367 = event shown="[1] \"QUIT\": Value Change" {
              selector: _ -> [_ _]
              dyn-events: _ -> [_ _]
              timeout: _ -> [_ _]
              tunnel: [_ w595] -> w591
              event "MAIN UI responsive? (F)": Value Change {
                n368 = event-data() -> ()  [unwired: 1 in, 1 out]
                n369 = Not(x="MAIN UI responsive? (F)") -> (.not. x?=w593:bool)
                n370 = property on="QUIT" class="Bool (strict)"("Visible"=w593) -> ()  [unwired: 2 in, 2 out]
              }
              event "QUIT": Value Change {
                w595 = TRUE  # QUIT
                n371 = event-data() -> ()  [unwired: 1 in, 1 out]
                n372 = property on="MAIN UI responsive? (F)" class="Bool (strict)"() -> ("Value"=w594:bool)  [unwired: 2 in, 2 out]
                n373 = case "If not responsive, QUIT all other VIs (including MAIN UI)." shown="False" w594 {
                  frame False {
                    n374 = control-ref of="This Application"() -> (w597:refnum<vi>)
                    n375 = property class="App"(reference=w597) -> (reference out=w599:refnum<vi>, error out=w600:errorcluster, "App.AllVIs"=w598:string[])  [unwired: 1 in]
                    n376 = Close Reference(reference=w599, error in (no error)=w600) -> (error out=w596:errorcluster)
                    n377 = for {
                      tunnel: w598 -> [w607] mode=indexing
                      tunnel: w596 -> [w602]
                      n378 = Open VI Reference(vi path=w607, error in (no error)=w602) -> (vi reference=w606:refnum<vi>, error out=w605:errorcluster)  [unwired: 4 in]
                      n379 = invoke class="VI" method="Abort VI"(reference=w606, error in=w605) -> (reference out=w604:refnum<vi>, error out=w603:errorcluster)  [unwired: 1 in, 1 out]
                      n380 = Close Reference(reference=w604, error in (no error)=w603) -> (error out=w601:errorcluster)
                      n381 = call <vilib>:"Clear Errors.vi"("error in (no error)"=w601) -> ()  [unwired: 6 in, 1 out]
                    }
                  }
                  frame True {
                    # "MAIN UI still responsive. Keep it running!"
                  }
                }
              }
            }
          }
        }
      }
    }
  }
  n382 = flat-sequence {
    tunnel: w4 -> [_]
    tunnel: w44 -> [w615]
    tunnel: [w615] -> w24
    tunnel: [w617] -> w26
    tunnel: w24 -> [w617]
    tunnel: w26 -> [w620]
    tunnel: [w620] -> w25
    tunnel: w17 -> [w619]
    tunnel: [w618] -> w15
    tunnel: w25 -> [w629]
    tunnel: [w628] -> w16
    tunnel: w15 -> [w628]
    tunnel: w16 -> [w633]
    frame #0 {
      # "Reset laser power"
      n383 = local write "piezo.active"(FALSE ("piezo.active")) -> ()
      n384 = call "GFG_core.vi"("Variable Name in"="Laser.Power" ("Variable Name"), "Variant in"=0.0, "Action"=enum16{"Init", "Set", "Get", "Clear"}."Set") -> ()  [unwired: 10 in, 7 out]
      n385 = call "GFG_core.vi"("Variable Name in"="Laser.Power.2" ("Variable Name"), "Variant in"=0.0, "Action"=enum16{"Init", "Set", "Get", "Clear"}."Set") -> ()  [unwired: 10 in, 7 out]
    }
    frame #1 {
      n386 = call "close modules.vi"("close FP?"=TRUE) -> ()  [unwired: 11 in]
    }
    frame #2 {
      n387 = Empty Array?(array=w619) -> (empty?=w618:bool)
      n388 = case "Write relative positions to inactive HS INIs" shown="False" w618 {
        tunnel: w619 -> [w627 _]
        tunnel: [w623 _] -> _
        tunnel: [w622 _] -> _
        frame False {
          w621 = "stage.control" ("Variable Name")
          w624 = string[] ["Xoffset", "Yoffset", "Zoffset"] ("Variables Names In")
          n389 = Index Array(array=w627) -> (element #1=w626:path, element #2=w625:path)  [unwired: 2 in]
          n390 = call "ReadSubsetofGFGandWritetoINI.vi"("Key Section (_)"=w621, "Variable Names In"=w624, "Path"=w626) -> ("error out"=w623:errorcluster)  [unwired: 8 in]
          n391 = call "ReadSubsetofGFGandWritetoINI.vi"("Key Section (_)"=w621, "Variable Names In"=w624, "Path"=w625) -> ("error out"=w622:errorcluster)  [unwired: 8 in]
        }
        frame True {
          # "Standalone version. No further action required."
        }
      }
    }
    frame #3 {
      n392 = Not(x=w629) -> (.not. x?=w630:bool)
      n393 = call "ReadGFGandWriteToINI.vi"() -> ("error out"=w631:errorcluster)  [unwired: 11 in]
      n394 = local write "QUIT"(w630) -> ()
      n395 = call "GFG_core.vi"("error in (no error)"=w631, "Action"=enum16{"Init", "Set", "Get"}."Init") -> ()  [unwired: 11 in, 7 out]
    }
    frame #4 {
      n396 = case shown="True" w633 {
        frame False {
          # "If this is not a standalone version, all DAQ devices will be reset when quitting the MAIN VI only. Don't do it here!"
        }
        frame True {
          # "If this is the standalone version, reset all DAQ devices."
          n397 = flat-sequence "Wait until SciScan stopped\nand reset all DAQ devices" {
            frame #0 {
              n398 = Wait (ms)(milliseconds to wait=u32 200) -> ()  [unwired: 1 out]
            }
            frame #1 {
              n399 = call "Reset_DAQ.vi"() -> ()  [unwired: 11 in, 1 out]
            }
          }
        }
      }
    }
  }
